vi "GetDigitalInputVals.vi"(8 "error in (no error)":errorcluster, 11 "SerialPortRef":T1) -> (0 "error out":errorcluster, 2 "All Digital Input Vals":bool[](array[boolean]), 3 "SerialPortRef 2":T1)   [LabVIEW 2015]
uses:
  <vilib>/Rock Robotics/WPI/SerialPort/WPI_SerialPortRef.ctl
panel:
  out "Receive":string
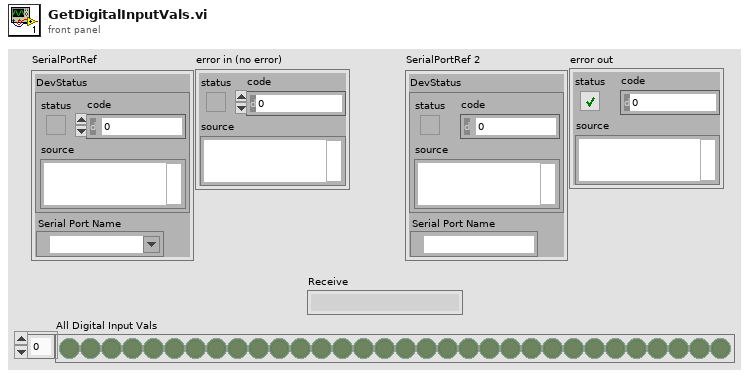
[diagram p1: front panel]
types:
  T1 = typedef "WPI_SerialPortRef.ctl" = cluster{"DevStatus":errorcluster, "Serial Port Name":refnum<visa-resource-name>}
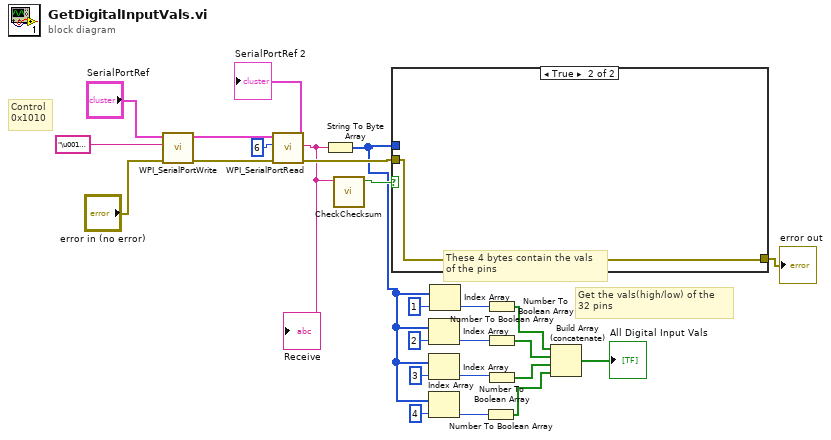
[diagram p0: block diagram]
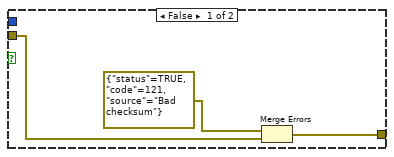
[diagram p2: hidden frame]
diagram:
  # "These 4 bytes contain the vals \nof the pins"
  # "Get the vals(high/low) of the \n32 pins"
  # "Control\n0x1010"
  n1 = call <vilib>:"WPI_SerialPortWrite.vi"("error in (no error)"="error in (no error)", "Buffer"="\u0010\u0010", "SerialPortRef"="SerialPortRef") -> ("error out"=w21:errorcluster, "SerialPortRef"=w22:T1)  [unwired: 6 in, 1 out]
  n2 = call <vilib>:"WPI_SerialPortRead.vi"("error in (no error)"=w21, "Num Bytes to Read"=u32 6, "SerialPortRef"=w22) -> ("error out"=w18:errorcluster, "Buffer"=w16:string, "SerialPortRef"=→"SerialPortRef 2":T1)  [unwired: 6 in]
  "Receive" <- w16
  n3 = String To Byte Array(string=w16) -> (unsigned byte array=w1:u8[])
  n4 = call "CheckChecksum.vi"("String"=w16) -> ("x = y?"=w15:bool)  [unwired: 10 in]
  n5 = case shown="True" w15 {
    tunnel: w1 -> [_ _]
    tunnel: w18 -> [w27 w29]
    tunnel: [w26 w29] -> w17
    frame False {
      n6 = Merge Errors(errorcluster {"status"=TRUE, "code"=121, "source"="Bad checksum"} ("error in"), w27) -> (w26:errorcluster)
    }
    frame True {
    }
  }
  "error out" <- w17
  n7 = Index Array(array=w1, index=2) -> (element=w9:u8)
  n8 = Index Array(array=w1, index=3) -> (element=w8:u8)
  n9 = Index Array(array=w1, index=4) -> (element=w7:u8)
  n10 = Index Array(array=w1, index=1) -> (element=w6:u8)
  n11 = Number To Boolean Array(number=w7) -> (Boolean array=w13:bool[])
  n12 = Number To Boolean Array(number=w6) -> (Boolean array=w10:bool[])
  n13 = Number To Boolean Array(number=w9) -> (Boolean array=w11:bool[])
  n14 = Number To Boolean Array(number=w8) -> (Boolean array=w12:bool[])
  n15 = Build Array (concatenate)(w10, w11, w12, w13) -> (→"All Digital Input Vals":bool[])
